vi "writeToXML.vi"(8 "error in (no error)":errorcluster, 11 "TCSPublicStatus in":refnum<class "TCSTcsStatus.lvclass">) -> (0 "error out":errorcluster, 2 "XML out":string="<tcsTCSStatus>\n  <tcsVersion/>\n  <accessMode>Operator</accessMode>\n  <azCurrentWrap>0</azCurrentWrap>\n  <heartbeat>0</heartbeat>\n  <inPositionIsTrue>false</inPositionIsTrue>\n  <m1CoverState>Open</m1CoverState>\n  <mountGuideMode>NoTrack</mountGuideMode>\n  <rotCurrentWrap>0</rotCurrentWrap>\n  <tcsHealth>GOOD</tcsHealth>\n  <tcsState>STANDBY</tcsState>\n  <currentTimes>\n    <lst>\n      <hours>0</hours>\n      <minutesTime>0</minutesTime>\n      <secondsTime>0</secondsTime>\n    </lst>\n    <time>1903-12-31T17:00:00.000-07:00</time>\n  </currentTimes>\n  <limits>\n    <moonProximity>\n      <distance_deg>0</distance_deg>\n      <proximityFlag>false</proximityFlag>\n    </moonProximity>\n    <sunProximity>\n      <distance_deg>0</distance_deg>\n      <proximityFlag>false</proximityFlag>\n    </sunProximity>\n    <zenith>\n      <currentZD_deg>0</currentZD_deg>\n      <elZenithLimit_deg>0</elZenithLimit_deg>\n      <inBlindSpotIsTrue>false</inBlindSpotIsTrue>\n      <timeToBlindSpot_min>0</timeToBlindSpot_min>\n      <timeToBlindSpotExit_min>0</timeToBlindSpotExit_min>\n    </zenith>\n    <airmass>0</airmass>\n    <currentTimeToObservable_min>0</currentTimeToObservable_min>\n    <currentTimeToUnobservable_min>0</currentTimeToUnobservable_min>\n    <timeToRotLimit_min>0</timeToRotLimit_min>\n    <timeToAzLimit_min>0</timeToAzLimit_min>\n  </limits>\n  <pointingPositions>\n    <azElError>\n      <azError>0</azError>\n      <elError>0</elError>\n    </azElError>\n    <currentAzEl>\n      <azimuth>\n        <degreesArc>0</degreesArc>\n        <minutesArc>0</minutesArc>\n        <secondsArc>0</secondsArc>\n      </azimuth>\n      <elevation>\n        <degreesAlt>90</degreesAlt>\n        <minutesArc>0</minutesArc>\n        <secondsArc>0</secondsArc>\n      </elevation>\n    </currentAzEl>\n    <currentHA>\n      <hours>0</hours>\n      <minutesTime>0</minutesTime>\n      <secondsTime>0</secondsTime>\n    </currentHA>\n    <currentRADec>\n      <declination>\n        <degreesDec>0</degreesDec>\n        <minutesArc>0</minutesArc>\n        <secondsArc>0</secondsArc>\n      </declination>\n      <equinoxPrefix>B</equinoxPrefix>\n      <equinoxYear>2000</equinoxYear>\n      <frame>FK4</frame>\n      <ra>\n        <hours>0</hours>\n        <minutesTime>0</minutesTime>\n        <secondsTime>0</secondsTime>\n      </ra>\n    </currentRADec>\n    <currentParAngle>0</currentParAngle>\n    <currentRotatorPositions>\n      <rotPA>0</rotPA>\n      <iaa>0</iaa>\n      <rotIPA>0</rotIPA>\n    </currentRotatorPositions>\n    <ObjectPA>\n      <EqPA>0</EqPA>\n      <AzPA>0</AzPA>\n    </ObjectPA>\n    <demandAzEl>\n      <azimuth>\n        <degreesArc>0</degreesArc>\n        <minutesArc>0</minutesArc>\n        <secondsArc>0</secondsArc>\n      </azimuth>\n      <elevation>\n        <degreesAlt>90</degreesAlt>\n        <minutesArc>0</minutesArc>\n        <secondsArc>0</secondsArc>\n      </elevation>\n    </demandAzEl>\n    <demandRADec>\n      <declination>\n        <degreesDec>0</degreesDec>\n        <minutesArc>0</minutesArc>\n        <secondsArc>0</secondsArc>\n      </declination>\n      <equinoxPrefix>B</equinoxPrefix>\n      <equinoxYear>2000</equinoxYear>\n      <frame>FK4</frame>\n      <ra>\n        <hours>0</hours>\n        <minutesTime>0</minutesTime>\n        <secondsTime>0</secondsTime>\n      </ra>\n    </demandRADec>\n    <demandRotatorPositions>\n      <rotPA>0</rotPA>\n    </demandRotatorPositions>\n    <targetName/>\n  </pointingPositions>\n  <OffsetStatus>\n    <offsetType>SIMPLE</offsetType>\n    <userOff1>0</userOff1>\n    <userOff2>0</userOff2>\n    <handsetOff1>0</handsetOff1>\n    <handsetOff2>0</handsetOff2>\n  </OffsetStatus>\n  <axesTrackMode>AzEl</axesTrackMode>\n  <inPositionAzIsTrue>false</inPositionAzIsTrue>\n  <inPositionElIsTrue>false</inPositionElIsTrue>\n  <inPositionRotIsTrue>false</inPositionRotIsTrue>\n  <externalTargetCfgCmdPreviewIsTrue>false</externalTargetCfgCmdPreviewIsTrue>\n</tcsTCSStatus>", 3 "TCSPublicStatus out":refnum<class "TCSTcsStatus.lvclass">)   [LabVIEW 2014, in "TCSDataDefinitions.lvlib" / "TCSPublicStatus.lvlib" / "TCSTcsStatus.lvclass"]
uses:
  TCSTcsStatus.lvclass
  TCSTcsStatus.lvclass/TCSTcsStatus.ctl
  CurrentTimes/CurrentTimes/CurrentTimes.lvclass
  Limits/Limits/Limits.lvclass
  PointingPositions/PointingPositions/PointingPositions.lvclass
  OffsetStatus/OffsetStatus/OffsetStatus.lvclass
  <userlib>/Common/XML/XMLGenerator/XMLGenerator.lvclass
panel:
  in  "ClassLabel":string="TCSTcsStatus"
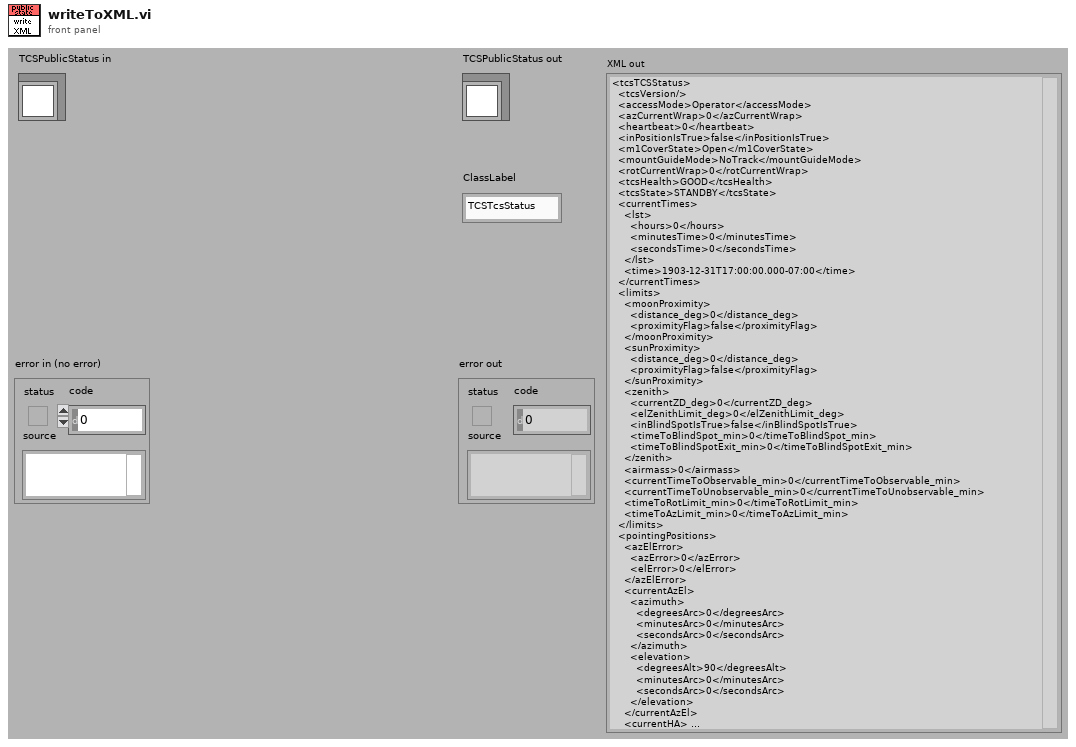
[diagram p1: front panel]
types:
  T1 = typedef "TCSDataDefinitions.lvlib/TCSPublicStatus.lvlib/AccessModeTypes.ctl" = enum16{"Operator", "Engineer"}
  T2 = typedef "TCSDataDefinitions.lvlib/TCSCommand.lvlib/CableWrapCommands.lvlib/WrapnumTypes.ctl" = enum16{"-1", "0", "1"}
  T3 = typedef "TCSDataDefinitions.lvlib/TCSPublicStatus.lvlib/M1CoverStateTypes.ctl" = enum16{"Open", "Closed", "PartiallyOpen"}
  T4 = typedef "TCSDataDefinitions.lvlib/TCSPublicStatus.lvlib/MountGuideModeTypes.ctl" = enum16{"NoTrack", "OpenLoop", "ClosedLoop"}
  T5 = typedef "TCSDataDefinitions.lvlib/TCSPublicStatus.lvlib/TCSHealthValues.ctl" = enum16{"GOOD", "WARNING", "BAD"}
  T6 = typedef "TCSDataDefinitions.lvlib/TCSPublicStatus.lvlib/TCSStateValues.ctl" = enum16{"STANDBY", "OFF", "ENABLED", "DISABLED", "FAULT"}
  T7 = typedef "TCSDataDefinitions.lvlib/TCSPublicStatus.lvlib/AxesTrackModeValues.ctl" = enum16{"AzEl", "All"}
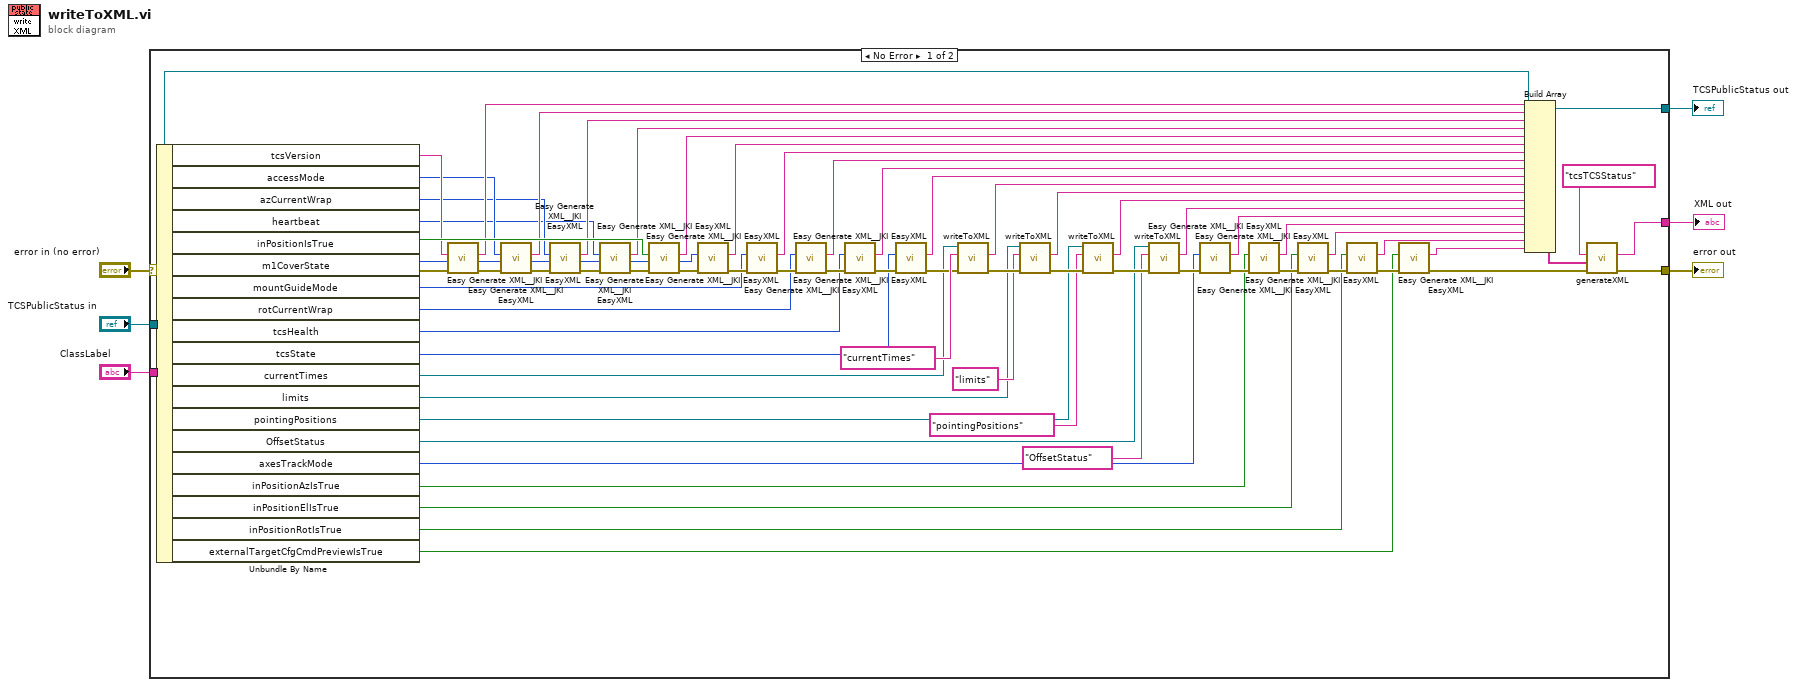
[diagram p0: block diagram]
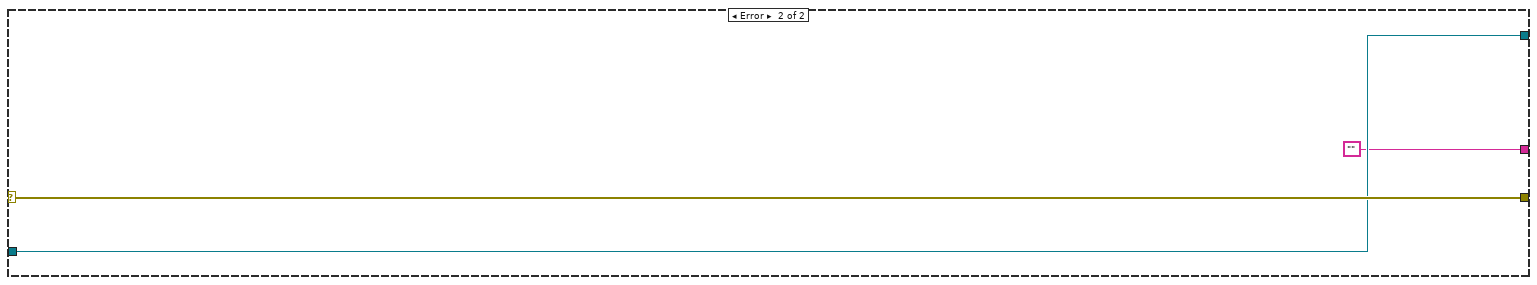
[diagram p2: hidden frame]
diagram:
  n1 = case shown="No Error" "error in (no error)" {
    selector: "error in (no error)" -> [w30 w75]
    tunnel: [w62 w75] -> w5
    tunnel: [w72 w74] -> w3
    tunnel: "TCSPublicStatus in" -> [w72 w74]
    tunnel: [w58 ""] -> w2
    tunnel: "ClassLabel" -> [_ _]
    frame No Error {
      n2 = Unbundle By Name(w72) -> ("tcsVersion"=w29:string, "accessMode"=w9:T1, "azCurrentWrap"=w8:T2, "heartbeat"=w7:u32, "inPositionIsTrue"=w32:bool, "m1CoverState"=w33:T3, "mountGuideMode"=w34:T4, "rotCurrentWrap"=w35:T2, "tcsHealth"=w36:T5, "tcsState"=w37:T6, "currentTimes"=w38:refnum<class "CurrentTimes.lvclass">, "limits"=w39:refnum<class "Limits.lvclass">, "pointingPositions"=w40:refnum<class "PointingPositions.lvclass">, "OffsetStatus"=w41:refnum<class "OffsetStatus.lvclass">, "axesTrackMode"=w44:T7, "inPositionAzIsTrue"=w42:bool, "inPositionElIsTrue"=w43:bool, "inPositionRotIsTrue"=w45:bool, "externalTargetCfgCmdPreviewIsTrue"=w46:bool)
      n3 = call <vilib>:"Easy Generate XML__JKI EasyXML.vi"("error in (no error)"=w30, "LabVIEW Data"=w29) -> ("error out"=w31:errorcluster, "XML String"=w28:string)  [unwired: 8 in]
      n4 = call <vilib>:"Easy Generate XML__JKI EasyXML.vi"("error in (no error)"=w31, "LabVIEW Data"=w9) -> ("error out"=w70:errorcluster, "XML String"=w10:string)  [unwired: 8 in]
      n5 = call <vilib>:"Easy Generate XML__JKI EasyXML.vi"("error in (no error)"=w70, "LabVIEW Data"=w8) -> ("error out"=w69:errorcluster, "XML String"=w11:string)  [unwired: 8 in]
      n6 = call <vilib>:"Easy Generate XML__JKI EasyXML.vi"("error in (no error)"=w69, "LabVIEW Data"=w7) -> ("error out"=w56:errorcluster, "XML String"=w12:string)  [unwired: 8 in]
      n7 = call <vilib>:"Easy Generate XML__JKI EasyXML.vi"("error in (no error)"=w56, "LabVIEW Data"=w32) -> ("error out"=w55:errorcluster, "XML String"=w13:string)  [unwired: 8 in]
      n8 = call <vilib>:"Easy Generate XML__JKI EasyXML.vi"("error in (no error)"=w55, "LabVIEW Data"=w33) -> ("error out"=w68:errorcluster, "XML String"=w14:string)  [unwired: 8 in]
      n9 = call <vilib>:"Easy Generate XML__JKI EasyXML.vi"("error in (no error)"=w68, "LabVIEW Data"=w34) -> ("error out"=w67:errorcluster, "XML String"=w15:string)  [unwired: 8 in]
      n10 = call <vilib>:"Easy Generate XML__JKI EasyXML.vi"("error in (no error)"=w67, "LabVIEW Data"=w35) -> ("error out"=w66:errorcluster, "XML String"=w16:string)  [unwired: 8 in]
      n11 = call <vilib>:"Easy Generate XML__JKI EasyXML.vi"("error in (no error)"=w66, "LabVIEW Data"=w36) -> ("error out"=w65:errorcluster, "XML String"=w17:string)  [unwired: 8 in]
      n12 = call <vilib>:"Easy Generate XML__JKI EasyXML.vi"("error in (no error)"=w65, "LabVIEW Data"=w37) -> ("error out"=w54:errorcluster, "XML String"=w18:string)  [unwired: 8 in]
      n13 = call-dynamic "writeToXML.vi"("error in (no error)"=w54, "Class Label"="currentTimes", "CurrentTimes in"=w38) -> ("error out"=w64:errorcluster, "XML out"=w19:string)  [unwired: 6 in, 1 out]
      n14 = call-dynamic "writeToXML.vi"("error in (no error)"=w64, "Class Label"="limits", "Limits in"=w39) -> ("error out"=w63:errorcluster, "XML out"=w20:string)  [unwired: 6 in, 1 out]
      n15 = call-dynamic "writeToXML.vi"("error in (no error)"=w63, "Class Label"="pointingPositions", "PointingPositions in"=w40) -> ("error out"=w53:errorcluster, "XML out"=w21:string)  [unwired: 6 in, 1 out]
      n16 = call-dynamic "writeToXML.vi"("ClassLabel"="OffsetStatus" ("Class Label"), "OffsetStatus in"=w41) -> ("XML out"=w22:string)  [unwired: 7 in, 2 out]
      n17 = call <vilib>:"Easy Generate XML__JKI EasyXML.vi"("error in (no error)"=w53, "LabVIEW Data"=w44) -> ("error out"=w52:errorcluster, "XML String"=w23:string)  [unwired: 8 in]
      n18 = call <vilib>:"Easy Generate XML__JKI EasyXML.vi"("error in (no error)"=w52, "LabVIEW Data"=w42) -> ("error out"=w51:errorcluster, "XML String"=w24:string)  [unwired: 8 in]
      n19 = call <vilib>:"Easy Generate XML__JKI EasyXML.vi"("error in (no error)"=w51, "LabVIEW Data"=w43) -> ("error out"=w50:errorcluster, "XML String"=w25:string)  [unwired: 8 in]
      n20 = call <vilib>:"Easy Generate XML__JKI EasyXML.vi"("error in (no error)"=w50, "LabVIEW Data"=w45) -> ("error out"=w49:errorcluster, "XML String"=w26:string)  [unwired: 8 in]
      n21 = call <vilib>:"Easy Generate XML__JKI EasyXML.vi"("error in (no error)"=w49, "LabVIEW Data"=w46) -> ("error out"=w47:errorcluster, "XML String"=w27:string)  [unwired: 8 in]
      n22 = Build Array(w28, w10, w11, w12, w13, w14, w15, w16, w17, w18, w19, w20, w21, w22, w23, w24, w25, w26, w27) -> (w71:string[])
      n23 = call <userlib>:"generateXML.vi"("error in"=w47, "childrenXML"=w71, "elementName"="tcsTCSStatus" ("Class Label")) -> ("error out"=w62:errorcluster, "XML out"=w58:string)  [unwired: 6 in, 1 out]
    }
    frame Error {
    }
  }
  "error out" <- w5
  "TCSPublicStatus out" <- w3
  "XML out" <- w2
